vi "Disconnect.vi"(8 "error in":errorcluster, 11 "SimulatedPS in":refnum<class "SimulatedPS.lvclass">) -> (0 "error out":errorcluster, 3 "SimulatedPS out":refnum<class "SimulatedPS.lvclass">)   [LabVIEW 2019, in "SimulatedPS.lvlib" / "SimulatedPS.lvclass"]
doc: "This disconnect routine is a must override from the Instrument Class\nChildren Classes are responsible for handling the override, but the parent class is an intermediary and must contain the override functions to maintain the rules for the method."
uses:
  Library/SimulatedPS.lvclass
  builds/Instruments/PowerSupply.lvlibp/Library/PowerSupply.lvclass
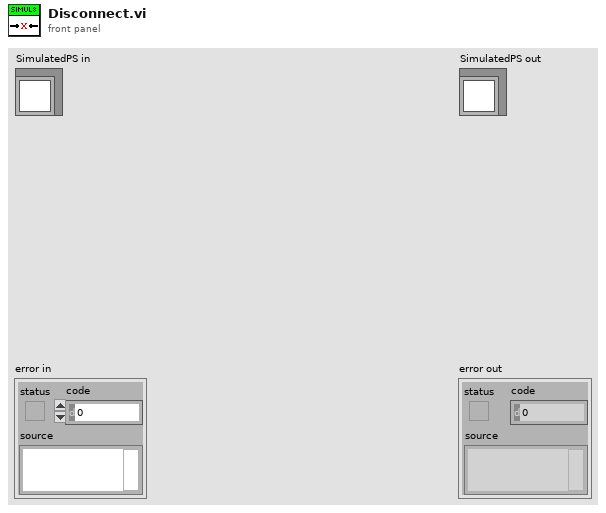
[diagram p1: front panel]
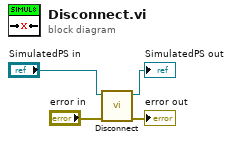
[diagram p0: block diagram]
diagram:
  n1 = call-parent "Disconnect.vi"("error in"="error in", "PowerSupply in"="SimulatedPS in") -> ("error out"=→"error out":errorcluster, "PowerSupply out"=→"SimulatedPS out":refnum<class "SimulatedPS.lvclass">)  [unwired: 8 in]
